vi "timekeeper epoch offset adjustment.vi"(0 "offset":fxp<+/-,64,64>) -> ()   [LabVIEW 2011, in "EPS_Timekeeper.lvlib"]
uses:
  <vilib>/addons/Electrical Power/Example Support/PMU/Time Keeper/EPS_Timekeeper.lvlib
  <vilib>/addons/Electrical Power/Example Support/PMU/Time Keeper/timekeeper time adjustment update toggle (g).vi
  <vilib>/addons/Electrical Power/Example Support/PMU/Time Keeper/timekeeper time adjustment offset (g).vi
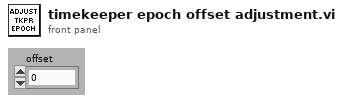
[diagram p1: front panel]
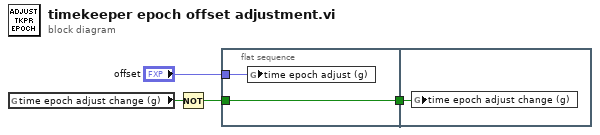
[diagram p0: block diagram]
diagram:
  n1 = global read "timekeeper time adjustment update toggle (g).vi" "time epoch adjust change (g)"() -> (w4:bool)
  n2 = Not(x=w4) -> (.not. x?=w3:bool)
  n3 = flat-sequence {
    tunnel: "offset" -> [w6]
    tunnel: w3 -> [w5]
    tunnel: [w5] -> w2
    tunnel: w2 -> [w7]
    frame #0 {
      n4 = global write "timekeeper time adjustment offset (g).vi" "time epoch adjust (g)"(w6) -> ()
    }
    frame #1 {
      n5 = global write "timekeeper time adjustment update toggle (g).vi" "time epoch adjust change (g)"(w7) -> ()
    }
  }
